vi "WaitScanMove.vi"(0 "Axis In":T1, 1 "Pause":refnum<vi>, 11 "error in (no error)":errorcluster, 12 "Stop":refnum<vi>) -> (4 "Axis Out":T1, 15 "error out":errorcluster)   [LabVIEW 2009]
doc: "Waits until axis is in position, an error occurs, or the stop control is activated in the caller VI. Pause will pause the current index until its value is changed back to inactive."
uses:
  typedefs/AxisSelect_Enum.ctl
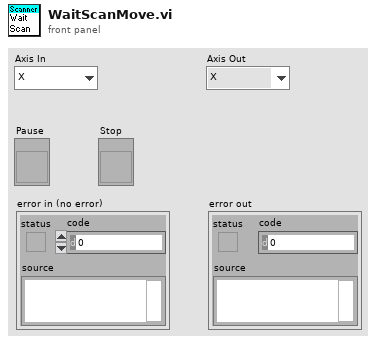
[diagram p1: front panel]
types:
  T1 = typedef "AxisSelect_Enum.ctl" = enum16{"X", "Y", "Z", "Axis Space"}
  T2 = typedef "DriveStatus_Cluster.ctl" = cluster{"In-position":bool, "Zero Speed":bool, "Enabled":bool, "Fault Disable":bool, "Ready":bool, "Start Index":bool, "Overtravel Exceeded":bool, "Up to Speed":bool, "Sequence Complete":bool}
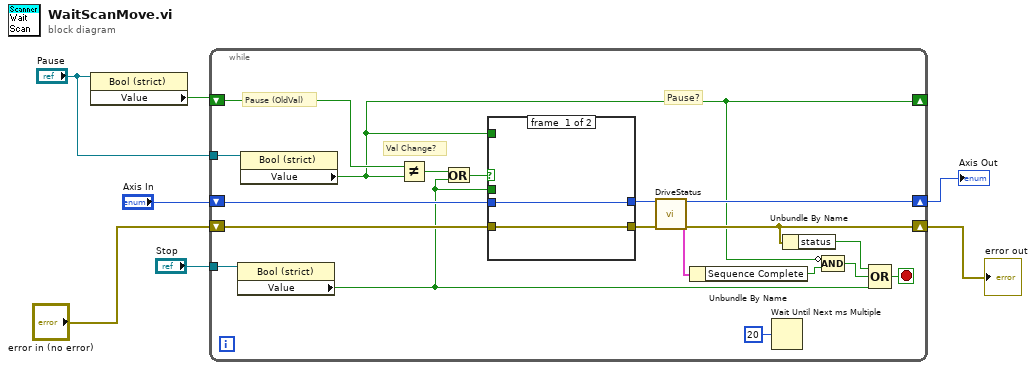
[diagram p0: block diagram]
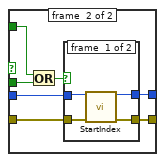
[diagram p2: hidden frame]
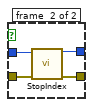
[diagram p3: hidden frame]
diagram:
  n1 = property class="Bool (strict)"(reference="Pause") -> ("Value"=w5:bool)  [unwired: 1 in, 2 out]
  n2 = while {
    shift-right: [w9] -> _
    shift-left: w5 -> [w12]
    shift-right: [w18] -> w6
    shift-left: "Axis In" -> [w24]
    tunnel: "Pause" -> [w22]
    tunnel: "Stop" -> [w21]
    shift-right: [w14] -> w2
    shift-left: "error in (no error)" -> [w15]
    stop <- w26 stop-if-true
    # "Val Change?"
    # "Pause (OldVal)"
    # "Pause?"
    n3 = property class="Bool (strict)"(reference=w21) -> ("Value"=w8:bool)  [unwired: 1 in, 2 out]
    n4 = property class="Bool (strict)"(reference=w22) -> ("Value"=w9:bool)  [unwired: 1 in, 2 out]
    n5 = Not Equal?(x=w12, y=w9) -> (x != y?=w10:bool)
    n6 = Or(x=w10, y=w8) -> (x .or. y?=w11:bool)
    n7 = case shown="True" w11 {
      tunnel: [w28 w35] -> w20
      tunnel: [w27 w34] -> w19
      tunnel: w24 -> [w28 w33]
      tunnel: w15 -> [w27 w32]
      tunnel: w9 -> [_ w31]
      tunnel: w8 -> [_ w29]
      frame #0 {
      }
      frame #1 {
        n8 = Or(x=w31, y=w29) -> (x .or. y?=w30:bool)
        n9 = case shown="False" w30 {
          tunnel: [w36 w43] -> w35
          tunnel: [w37 w42] -> w34
          tunnel: w33 -> [w39 w41]
          tunnel: w32 -> [w38 w40]
          frame #0 {
            n10 = call "StartIndex.vi"("Axis In (Axis Space)"=w39, "error in (no error)"=w38) -> ("Axis Out"=w36:T1, "error out"=w37:errorcluster)  [unwired: 12 in]
          }
          frame #1 {
            n11 = call "StopIndex.vi"("Axis In (Axis Space)"=w41, "error in (no error)"=w40) -> ("Axis Out"=w43:T1, "error out"=w42:errorcluster)  [unwired: 12 in]
          }
        }
      }
    }
    n12 = call "DriveStatus.vi"("Axis In"=w20, "error in (no error)"=w19) -> ("Axis Out"=w18:T1, "Status"=w17:T2, "error out"=w14:errorcluster)  [unwired: 11 in]
    n13 = Unbundle By Name(w17) -> ("Sequence Complete"=w16:bool)
    n14 = Wait Until Next ms Multiple(millisecond multiple=u32 20) -> ()  [unwired: 1 out]
    n15 = Unbundle By Name(w14) -> ("status"=w13:bool)
    n16 = Compound Arithmetic op=AND(invert w9, w16) -> (w23:bool)
    n17 = Compound Arithmetic op=OR(w13, w23, w8) -> (w26:bool)
  }
  "Axis Out" <- w6
  "error out" <- w2
